vi "TestSubVI.vi"(1 "x":dbl=5.0, 2 "y":dbl=5.0) -> (0 "y+x^2":dbl)   [LabVIEW 2020]
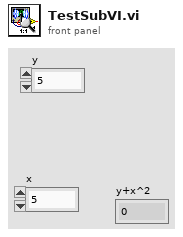
[diagram p1: front panel]
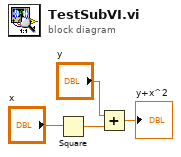
[diagram p0: block diagram]
diagram:
  n1 = Square(x="x") -> (x^2=w2:dbl)
  n2 = Add(x="y", y=w2) -> (x+y=→"y+x^2":dbl)
